vi "PROJECTE OCELL FINAL 0.1.vi"() -> ()   [LabVIEW 2020]
uses:
  <vilib>/numeric/Random Number (Range) DBL.vi
  <vilib>/MakerHub/LINX/Public/Utilities/Open Serial.vi
  <vilib>/MakerHub/LINX/LMH-LINX.lvlib
  <vilib>/MakerHub/LINX/Public/Sensors/Distance/Ultrasonic/Ultrasonic.lvlib
panel:
  out "String":string="HEU GUANYAT !!!"
  in  "TEMPS D'ESPERA":i32=30
  in  "JUGADOR 2":dbl(slide)=5.1020408163265305 scale=0.0..100.0
  in  "JUGADOR 1":dbl(slide)=3.0612244897959187 scale=0.0..100.0
  in  "Velocitat de moviment":u32=100
  out "Error Out":errorcluster={"status"=TRUE, "code"=54, "source"="TCP Open Connection in LMH-LINX.lvlib:Device.lvlib:TCP Open.vi->LMH-LINX.lvlib:Device.lvlib:Initialize Device.vi->LMH-LINX.lvlib:Initialize.vi->LMH-LINX.lvlib:Open Serial.vi->PROJECTE OCELL jugador esquerra.vi"}
  in  "Control d'aturada":bool
  in  "DI Channel":u8
  out "Device Name":string
  in  "Error In":errorcluster
  in  "Baud Rate Override":u32=9600
  in  "Serial Port":refnum<visa-resource-name>="N/A"
  out "Monitor":cluster{dbl[], dbl[]}[](graph)=[{[0.99, 0.985, 0.98, 0.975, 0.86, 0.88, 0.9, 0.92, 0.94, 0.96, 0.98, 1.0, 0.94, 0.96, 0.98, 0.86], [0.0, 1.0, 2.0, 3.0, 4.0, 4.0, 4.0, 4.0, 4.0, 4.0, 4.0, 4.0, 3.0, 2.0, 1.0, 4.5]}, {[0.0, 0.0, 0.0, 0.02, 0.02, 0.02, 0.04, 0.04, 0.06, -0.06, -0.04, -0.04, -0.02, -0.02, -0.02], [2.0, 4.0, 3.0, 4.0, 5.0, 3.0, 5.0, 6.0, 6.0, 6.0, 6.0, 5.0, 5.0, 3.0, 4.0]}, {[-0.99, -0.985, -0.98, -0.975, -0.86, -0.88, -0.9, -0.92, -0.94, -0.96, -0.98, -1.0, -0.94, -0.96, -0.98, -0.86], [0.0, 1.0, 2.0, 3.0, 4.0, 4.0, 4.0, 4.0, 4.0, 4.0, 4.0, 4.0, 3.0, 2.0, 1.0, 4.5]}]
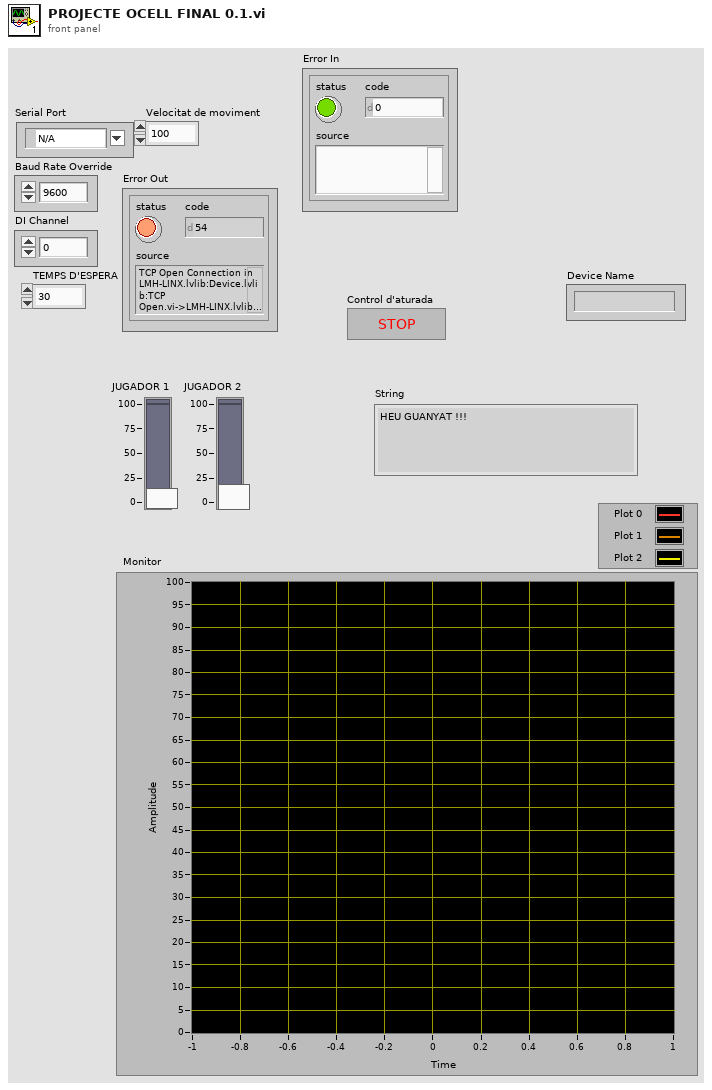
[diagram p1: front panel]
types:
  T1 = typedef "LMH-LINX.lvlib/LINX Ref.ctl" = cluster{"IO":T2, "Interface":T3, "LINX Device Config":T4}
  T2 = typedef "LMH-LINX.lvlib/Platform.ctl" = enum16{"Remote", "Local"}
  T3 = typedef "LMH-LINX.lvlib/Interface.ctl" = enum16{"Serial", "TCP"}
  T4 = typedef "LMH-LINX.lvlib/Device.lvlib/LINX Device Config.ctl" = cluster{"Interface":T3, "COM Port":refnum<visa-resource-name>, "TCP Configuration":T5, "Device Family":u8, "Device ID":u8, "Device Name":string, "TCP Ref":refnum<k5>, "Channels":T6}
  T5 = typedef "LMH-LINX.lvlib/Device.lvlib/TCP Config.ctl" = cluster{"IP Address":string, "Port":u16}
  T6 = typedef "LMH-LINX.lvlib/Channels.ctl" = cluster{"DI":u8[], "DO":u8[], "AI":u8[], "AO":u8[], "PWM":u8[], "QE":u8[], "UART":u8[], "I2C 2":u8[], "SPI":u8[], "CAN":u8[], "Servo":u8[], "AI Ref (V)":dbl, "AI Resolution (Bits)":u8, "AO Ref (V)":dbl, "AO Resolution (Bits)":u8}
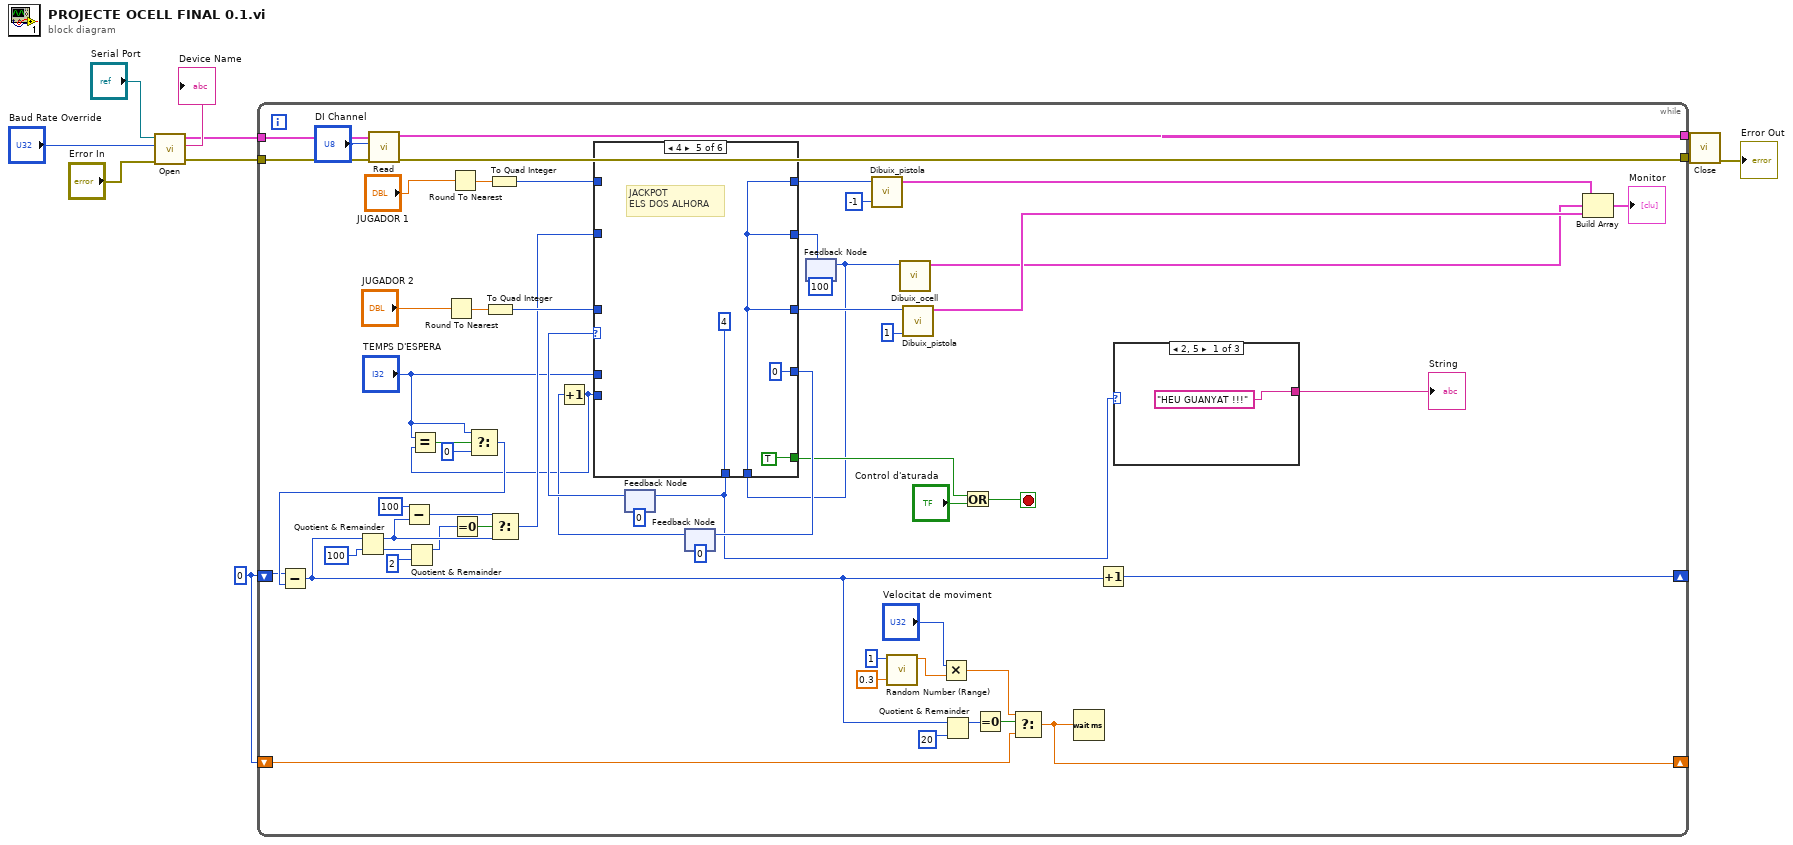
[diagram p0: block diagram]
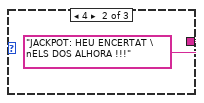
[diagram p2: hidden frame]
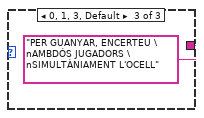
[diagram p3: hidden frame]
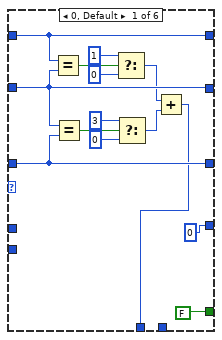
[diagram p4: hidden frame]
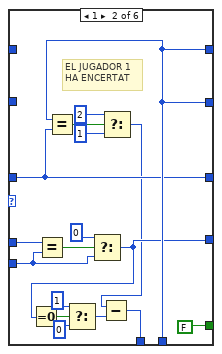
[diagram p5: hidden frame]
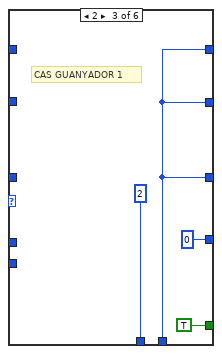
[diagram p6: hidden frame]
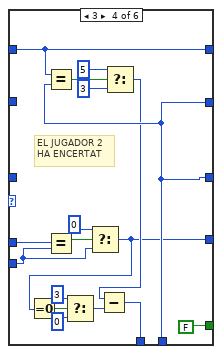
[diagram p7: hidden frame]
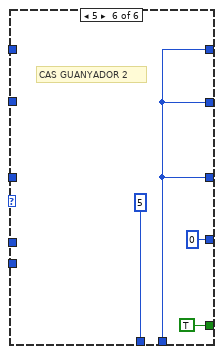
[diagram p8: hidden frame]
diagram:
  w1 = 0
  n1 = call-poly <vilib>:"Open.vi"("Error In"="Error In", "Baud Rate Override"="Baud Rate Override", "Serial Port"="Serial Port") -> ("Error Out"=w6:errorcluster, "Device Name"=→"Device Name":string, "LINX Resource"=w7:T1)  [unwired: 6 in]
  n2 = while {
    tunnel: w7 -> [w69]
    tunnel: w6 -> [w68]
    tunnel: [w65] -> w5
    tunnel: [w64] -> w4
    shift-right: [w36] -> _
    shift-left: w1 -> [w34]
    shift-right: [w21] -> _
    shift-left: w1 -> [w22]
    stop <- w44 stop-if-true
    n3 = call <vilib>:"Read.vi"("Error In"=w68, "DI Channel"="DI Channel", "LINX Resource"=w69) -> ("Error Out"=w64:errorcluster, "LINX Resource"=w65:T1)  [unwired: 5 in, 2 out]
    n4 = Round To Nearest(number="JUGADOR 2") -> (nearest integer value=w53:dbl)
    n5 = Round To Nearest(number="JUGADOR 1") -> (nearest integer value=w55:dbl)
    n6 = To Quad Integer(1:w53) -> (0:w50:i64)
    n7 = To Quad Integer(1:w55) -> (0:w54:i64)
    n8 = feedback #1(0 ("f")) -> (w49:i32)
    n9 = feedback #2(0 ("t")) -> (w37:i32)
    n10 = Increment(x=w37) -> (x+1=w32:i32)
    n11 = Equal?(x="TEMPS D'ESPERA", y=w32) -> (x = y?=w39:bool)
    n12 = Select(t="TEMPS D'ESPERA", s=w39, f=0) -> (s? t:f=w35:i32)
    n13 = Subtract(x=w34, y=w35) -> (x-y=w30:i32)
    n14 = Quotient & Remainder(x=w30, y=100) -> (x-y*floor(x/y)=w61:i32, floor(x/y)=w58:i32)
    n15 = Subtract(x=100 ("y"), y=w61) -> (x-y=w60:i32)
    n16 = Quotient & Remainder(x=w58, y=2) -> (x-y*floor(x/y)=w56:i32)  [unwired: 1 out]
    n17 = Equal To 0?(x=w56) -> (x = 0?=w57:bool)
    n18 = Select(t=w60, s=w57, f=w61) -> (s? t:f=w41:i32)
    n19 = feedback #3(100) -> (w14:i32)
    n20 = case shown="4" w49 {
      tunnel: w54 -> [w86 _ _ w121 _ _]
      tunnel: [w86 w100 w106 w121 w127 w131] -> w16
      tunnel: w41 -> [w79 _ _ _ _ _]
      tunnel: [w79 w100 w106 w120 w127 w131] -> w52
      tunnel: w14 -> [_ w100 w106 w120 w127 w131]
      tunnel: w50 -> [w78 w99 _ _ _ _]
      tunnel: [w78 w99 w106 w120 w127 w131] -> w18
      tunnel: [w75 w91 2 ("f") w111 4 ("f") 5 ("f")] -> w12
      tunnel: [FALSE FALSE TRUE FALSE TRUE TRUE] -> w40
      tunnel: w32 -> [_ w95 _ w110 _ _]
      tunnel: [0 ("t") w93 0 ("t") w108 0 ("t") 0 ("t")] -> w43
      tunnel: "TEMPS D'ESPERA" -> [_ w94 _ w109 _ _]
      frame 0, Default {
        n21 = Equal?(x=w86, y=w79) -> (x = y?=w85:bool)
        n22 = Equal?(x=w79, y=w78) -> (x = y?=w82:bool)
        n23 = Select(t=1, s=w85, f=0) -> (s? t:f=w76:i32)
        n24 = Select(t=3, s=w82, f=0) -> (s? t:f=w77:i32)
        n25 = Add(x=w76, y=w77) -> (x+y=w75:i32)
      }
      frame 1 {
        # "EL JUGADOR 1\nHA ENCERTAT"
        n26 = Equal?(x=w94, y=w95) -> (x = y?=w97:bool)
        n27 = Equal?(x=w100, y=w99) -> (x = y?=w103:bool)
        n28 = Select(t=0, s=w97, f=w95) -> (s? t:f=w93:i32)
        n29 = Equal To 0?(x=w93) -> (x = 0?=w89:bool)
        n30 = Select(t=1, s=w89, f=0 ("t")) -> (s? t:f=w90:i32)
        n31 = Select(t=2, s=w103, f=1) -> (s? t:f=w92:i32)
        n32 = Subtract(x=w92, y=w90) -> (x-y=w91:i32)
      }
      frame 2 {
        # "CAS GUANYADOR 1"
      }
      frame 3 {
        # "EL JUGADOR 2\nHA ENCERTAT"
        n33 = Equal?(x=w121, y=w120) -> (x = y?=w124:bool)
        n34 = Equal?(x=w109, y=w110) -> (x = y?=w118:bool)
        n35 = Select(t=0, s=w118, f=w110) -> (s? t:f=w108:i32)
        n36 = Equal To 0?(x=w108) -> (x = 0?=w115:bool)
        n37 = Select(t=3, s=w115, f=0 ("t")) -> (s? t:f=w116:i32)
        n38 = Select(t=5, s=w124, f=3) -> (s? t:f=w112:i32)
        n39 = Subtract(x=w112, y=w116) -> (x-y=w111:i32)
      }
      frame 4 {
        # "JACKPOT\nELS DOS ALHORA"
      }
      frame 5 {
        # "CAS GUANYADOR 2"
      }
    }
    n40 = feedback-in #1(w12) -> ()
    n41 = feedback-in #2(w43) -> ()
    n42 = feedback-in #3(w52) -> ()
    n43 = call "Dibuix_pistola.vi"("Esquerra/Dreta (-1/1)"=-1, "Posició Y"=w16) -> ("Dibuix pistola"=w20:cluster{dbl[], dbl[]})  [unwired: 9 in]
    n44 = call-poly <vilib>:"Random Number (Range).vi"("lower bound (0)"=0.3, "upper bound (100)"=u64 1) -> ("number"=w24:dbl)  [unwired: 9 in]
    n45 = call "Dibuix_ocell.vi"("Posició Y"=w14) -> ("Dibuix pistola"=w13:cluster{dbl[], dbl[]})  [unwired: 10 in]
    n46 = call "Dibuix_pistola.vi"("Esquerra/Dreta (-1/1)"=1, "Posició Y"=w18) -> ("Dibuix pistola"=w17:cluster{dbl[], dbl[]})  [unwired: 9 in]
    n47 = Multiply(x="Velocitat de moviment", y=w24) -> (x*y=w23:dbl)
    n48 = Quotient & Remainder(x=w30, y=20 ("f")) -> (x-y*floor(x/y)=w29:i32)  [unwired: 1 out]
    n49 = Or(x=w40, y="Control d'aturada") -> (x .or. y?=w44:bool)
    n50 = Equal To 0?(x=w29) -> (x = 0?=w28:bool)
    n51 = Select(t=w23, s=w28, f=w22) -> (s? t:f=w21:dbl)
    n52 = Wait (ms)(milliseconds to wait=w21) -> ()  [unwired: 1 out]
    n53 = Increment(x=w30) -> (x+1=w36:i32)
    n54 = case shown="2, 5" w12 {
      tunnel: ["HEU GUANYAT !!!" "JACKPOT: HEU ENCERTAT \nELS DOS ALHORA !!!" "PER GUANYAR, ENCERTEU \nAMBDÓS JUGADORS \nSIMULTÀNIAMENT L'OCELL"] -> w11
      frame 2, 5 {
      }
      frame 4 {
      }
      frame 0, 1, 3, Default {
      }
    }
    "String" <- w11
    n55 = Build Array(w20, w13, w17) -> (→"Monitor":cluster{dbl[], dbl[]}[])
  }
  n56 = call <vilib>:"Close.vi"("Error In"=w4, "LINX Resource"=w5) -> ("Error Out"=→"Error Out":errorcluster)  [unwired: 9 in]
